vi "Accelerator_v2.001.vi"() -> ()   [LabVIEW 2012]
doc: "Acquire Accelerator Data"
uses:
  <instrlib>/niScope/Controls/niScope vertical coupling.ctl
  <instrlib>/niScope/Controls/niScope trigger slope.ctl
  <instrlib>/niScope/Controls/niScope trigger coupling.ctl
  <instrlib>/niScope/Controls/niScope trigger window mode.ctl
  <instrlib>/niScope/Controls/niScope trigger source.ctl
  Array_Defctl.ctl
  <vilib>/Utility/error.llb/DialogType.ctl
  Database2.0/Public API/Dust_Event.ctl
  Database2.0/Public API/Signal.ctl
  Database2.0/Private/Role ID.ctl
  Database2.0/Private/Hardware ID.ctl
  Database2.0/Private/Estimate_source.ctl
  Database2.0/Private/PSU updated.vi
  <vilib>/addons/database/Connection.llb/Conn Execute.vi
  <vilib>/addons/database/Recordset.llb/Rec Fetch Recordset Data (R).vi
  <vilib>/addons/database/Recordset.llb/Rec Destroy - Connection.vi
  <instrlib>/niScope/Configure/Trigger/niScope Configure Trigger Edge.vi
  <instrlib>/niScope/Configure/Trigger/niScope Configure Trigger Hysteresis.vi
  <instrlib>/niScope/Configure/Trigger/niScope Configure Trigger Window.vi
  <instrlib>/niScope/Configure/Trigger/niScope Configure Trigger Immediate.vi
  <instrlib>/niScope/Acquire/Fetch/niScope Multi Fetch Cluster.vi
  <vilib>/Analysis/baseanly.llb/Mean (DBL).vi
  <vilib>/Utility/file.llb/Write To Spreadsheet File (string).vi
  <vilib>/addons/database/_DB Variant To Data/Database Variant To Data.xnode
  <vilib>/Analysis/NI_AALBase.lvlib
  <vilib>/addons/database/NI_Database_API.lvlib
panel:
  out "?":cluster{dbl, dbl}(knob)={0.0549, 2.0} scale=10.0..0.01
  in  "Ideal Time (Cursor)":dbl=2.0 step=0.01 format="%_2f"
  out "Time Between Triggers":dbl
  out "Average Frequency":dbl format="%#_4g"
  in  "Write to Database?":bool=TRUE
  out "output cluster":T1
  out "error out 4":errorcluster
  out "error out 3":errorcluster
  out "# elements in queue":i32
  out "Stop condition":bool=TRUE
  in  "Limit":dbl
  in  "Limit Triggers":bool
  out "Metadata Path":path=path "G:/default/20120619111009.csv"
  out "created path":path=path "G:/default"
  in  "Write Metadata?":bool
  out "Acquisition #":i32
  out "Numeric":i32=92364
  out "error out 2":errorcluster
  out "Calibration":dbl=24700000000000.0
  in  "WFM Tag":string="trace"
  in  "Location":string="G:\\default"
  in  "Write Raw File?":bool
  out "Saving Raw File...":path=path "G:/2012_06_13_verify_timestamp_labview/trace00000"
  out "Array":T2=["Dev1", "Dev2"]
  in  "Debug Mode\n(Confusing)":bool
  out "Mass":dbl format="%#_3g"
  out "Multi Plot 2":cluster{dbl[], dbl[]}(graph) caption="Multi Plot"
  in  "Acceleration Voltage (MV)":dbl=2.0 format="%_2g"
  out "Charge":dbl format="%#_3g"
  out "Velocity (Est.)":dbl format="%#_6f"
  out "Final Detector (CH3)":waveform(dbl)(graph)={"t0"=timestamp(0 s since 1904-01-01), "dt"=1e-07, "Y"=[]}
  out "Charge Detector/PSU gate (CH2)":waveform(dbl)(graph)={"t0"=timestamp(0 s since 1904-01-01), "dt"=1e-07, "Y"=[]}
  out "Velocity Detectors (CH0 & CH1)":waveform(dbl)[](graph)
  out "Actual Sample Rate":dbl=10000000.0 format="%.0p"
  in  "Reference Position (%)":dbl=40.0 caption="Ref Position" format="%.1f"
  in  "Trigger":T3(tab)=enum."Edge"
  in  "Trigger Source Edge 2":T4="2" caption="Source"
  in  "Trigger Source Edge":T4="0" caption="Source"
  in  "Coupling":T5=1 items=["AC"=0, "DC"=1, "HF Reject"=3, "LF Reject"=4, "AC Plus HF Reject"=1001]
  in  "Slope":T6 caption="Trigger Slope"
  in  "Level":dbl=1.0 caption="Trigger Level" step=0.001 format="%.3f"
  in  "Delay":dbl caption="Trigger Delay" format="%.4p"
  in  "Trigger Source Window 2":T4="0" caption="Source"
  in  "Trigger Source Window":T4="0" caption="Source"
  in  "Window Mode":T7=1
  in  "Delay":dbl caption="Trigger Delay" format="%.4f"
  in  "Low Level":dbl=-0.12 format="%.2f"
  in  "High Level":dbl format="%.2f"
  in  "Window Coupling":T5=1 caption="Coupling" items=["AC"=0, "DC"=1, "HF Reject"=3, "LF Reject"=4, "AC Plus HF Reject"=1001]
  in  "Hysteresis Source Trigger 2":T4="3" caption="Source"
  in  "Hysteresis Source Trigger":T4="1" caption="Source"
  in  "Hysteresis":dbl format="%.2f"
  in  "Delay":dbl caption="Trigger Delay" format="%.4f"
  in  "Slope":T6 caption="Trigger Slope"
  in  "Hysteresis Coupling":T5=1 caption="Coupling" items=["AC"=0, "DC"=1, "HF Reject"=3, "LF Reject"=4, "AC Plus HF Reject"=1001]
  in  "Level":dbl=0.05 caption="Trigger Level" format="%.2f"
  in  "Vertical Coupling":T8=1 items=["AC", "DC", "Ground"]
  in  "Probe Attenuation":dbl=1.0 format="%.1f"
  in  "Vertical Offset":dbl format="%.4f"
  in  "Vertical Range":dbl=5.0 caption="Vertical Range (V)" format="%.2f"
  in  "Bandwidth":dbl=-1.0 format="%.2f"
  in  "Min Record Length":i32=100000 caption="Min. Record Length"
  in  "Min Sample Rate":dbl=80000000.0 caption="Min. Sample Rate" step=1000000.0 format="%.2p"
  out "Actual Record Length":i32=100000
  in  "stop":bool=TRUE
  out "error out":errorcluster={"status"=FALSE, "code"=0, "source"="No Error"} {"code" format="%.0x"}
  # "File Parameters"
  # "Error Handling"
  # "Horizontal"
  # "Vertical"
  # "Channel"
  # "Trigger"
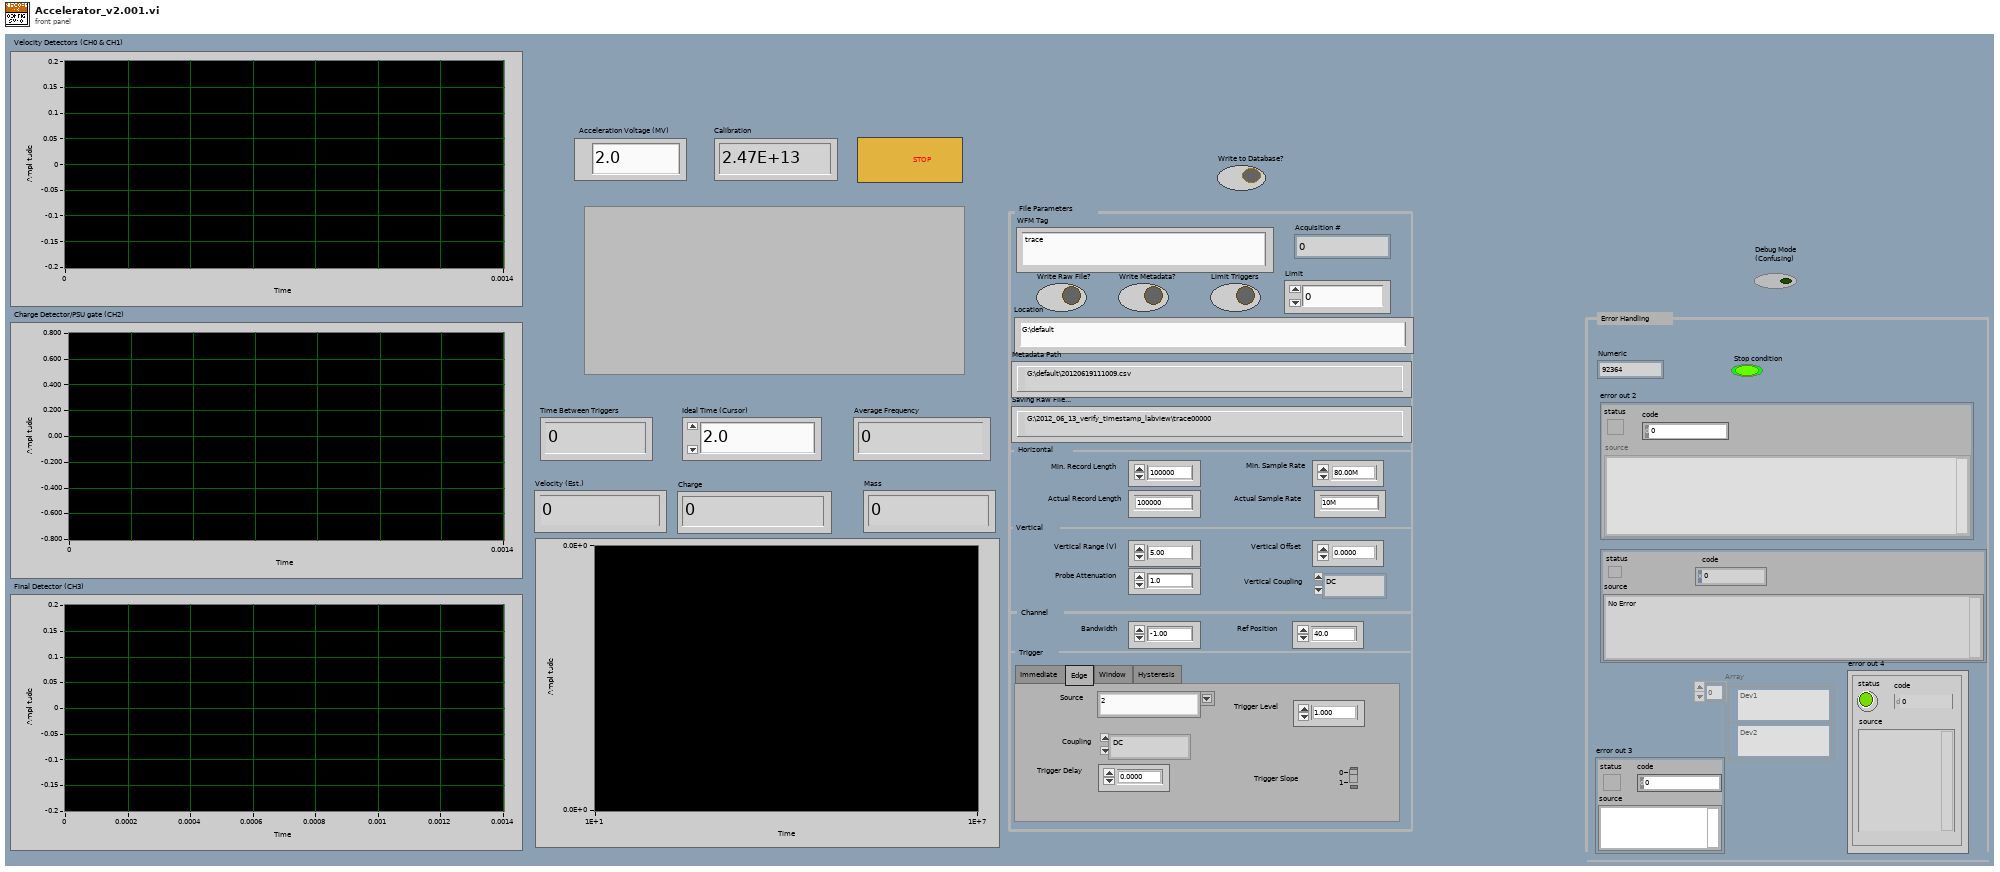
[diagram p1: front panel]
types:
  T1 = cluster{"File Path Control":path, "Array":waveform(dbl)[]}
  T2 = typedef "Array_Defctl.ctl" = refnum<k15>[]
  T3 = enum32{"Immediate", "Edge", "Window", "Hysteresis"}
  T4 = typedef "niScope trigger source.ctl" = string
  T5 = typedef "niScope trigger coupling.ctl" = u16
  T6 = typedef "niScope trigger slope.ctl" = i32
  T7 = typedef "niScope trigger window mode.ctl" = i32
  T8 = typedef "niScope vertical coupling.ctl" = i32
  T9 = typedef "DialogType.ctl" = u16
  T10 = typedef "NI_Database_API.lvlib/Conn ObjectReference.ctl" = refnum<k1>
  T11 = typedef "NI_Database_API.lvlib/Rec ObjectReference.ctl" = refnum<k1>
  T12 = cluster{"Integer Timestamp":dbl, "Max Velocity":dbl, "Min Velocity":dbl}
  T13 = cluster{"first point time":dbl, "xIncrement":dbl, "Waveforms":dbl[]}[]
  T14 = typedef "Dust_Event.ctl" = cluster{"Time Stamp":timestamp, "Velocity":sgl, "Mass":sgl, "Charge":sgl, "Radius":sgl, "Array":T15[], "Dust Event ID":i64, "Passed_3rd_Detector":bool, "Estimate Source":T18, "Estimate Quality":sgl}
  T15 = typedef "Signal.ctl" = cluster{"Signal ID":i64, "Time Stamp":timestamp, "Dust Event ID":i64, "Role ID":T16, "Data":sgl[], "Signal Length":i32, "dt":sgl, "Offset":dbl, "Hardware ID":T17}
  T16 = typedef "Role ID.ctl" = enum16{"First_Detector", "Second_Detector", "Third_Detector", "LeCroy_CH1", "LeCroy_CH2", "LeCroy_CH3", "LeCroy_CH4", "PSU"}
  T17 = typedef "Hardware ID.ctl" = enum16{"Unknown", "CSA 1", "CSA 2", "CSA 3", "CSA 4", "CSA 5", "CSA 6"}
  T18 = typedef "Estimate_source.ctl" = i8
  T19 = cluster{"relativeInitialX":dbl, "xIncrement":dbl, "wfm":dbl[]}[]
  T20 = cluster{"first point time":dbl, "xIncrement":dbl, "Waveforms":dbl[]}
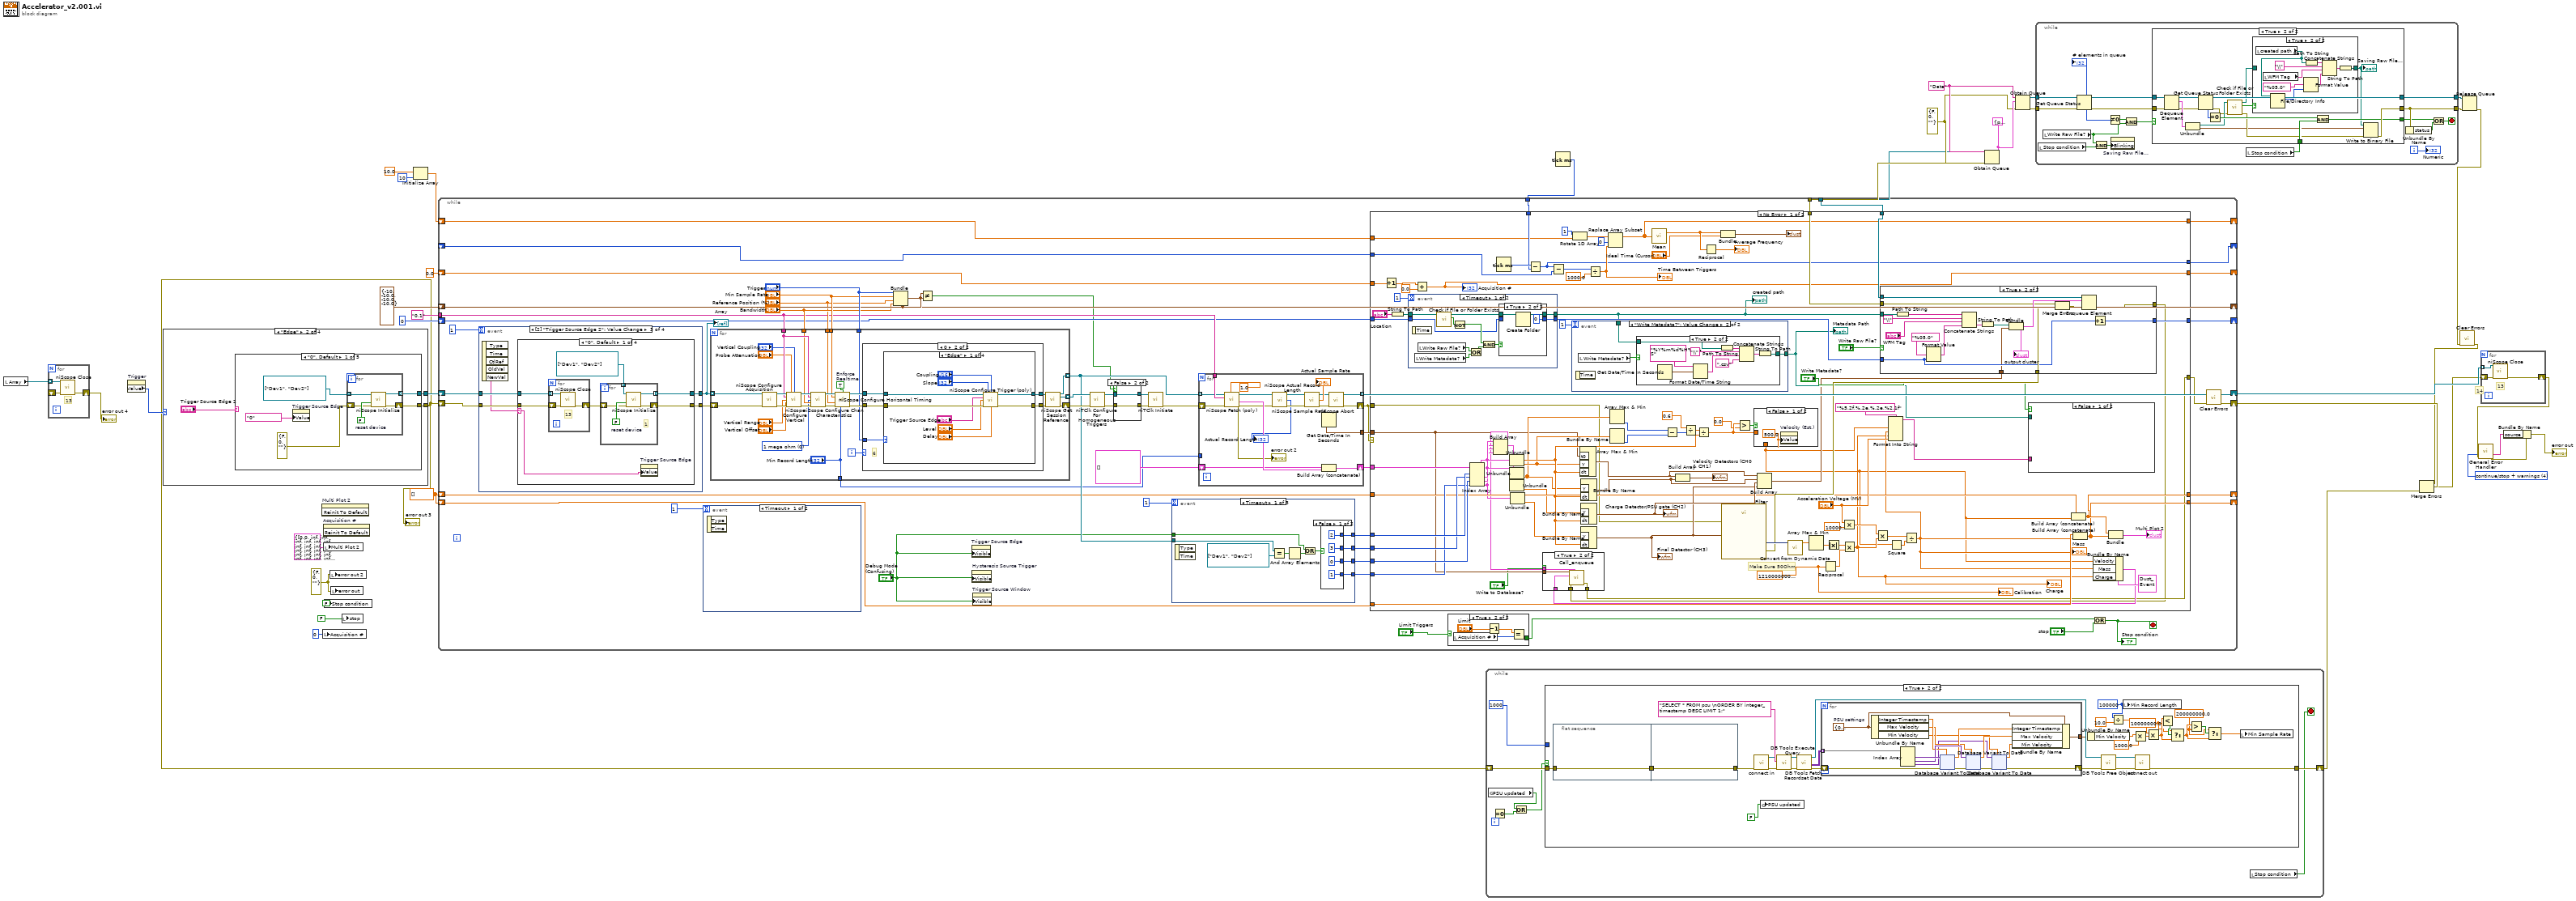
[diagram p0: block diagram]
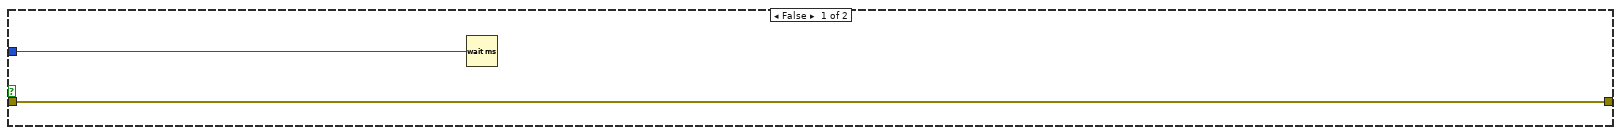
[diagram p2: hidden frame]
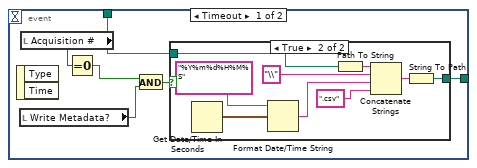
[diagram p4: hidden frame]
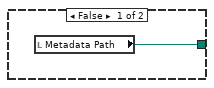
[diagram p5: hidden frame]
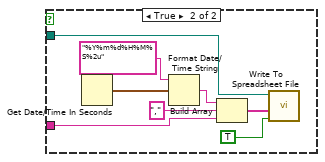
[diagram p7: hidden frame]
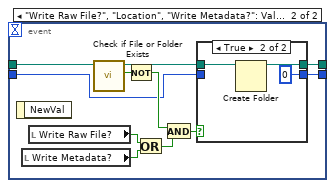
[diagram p9: hidden frame]
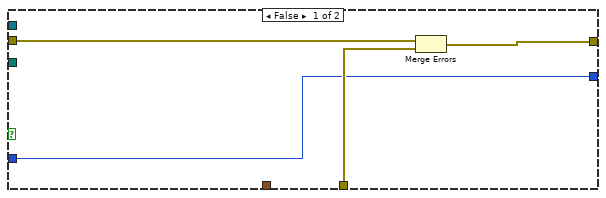
[diagram p11: hidden frame]
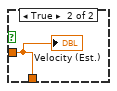
[diagram p12: hidden frame]
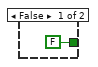
[diagram p14: hidden frame]
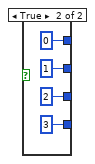
[diagram p15: hidden frame]
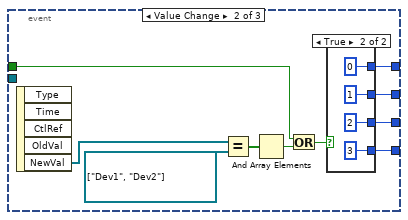
[diagram p16: hidden frame]
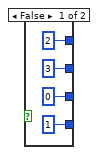
[diagram p17: hidden frame]
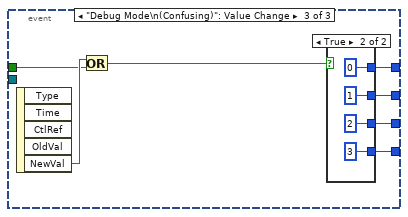
[diagram p18: hidden frame]
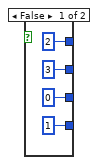
[diagram p19: hidden frame]
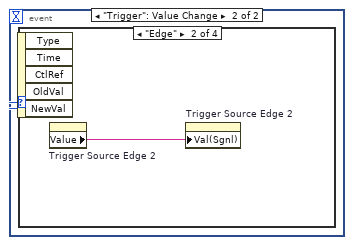
[diagram p20: hidden frame]
diagram:
  w4 = dbl[] []
  w11 = errorcluster {"status"=FALSE, "code"=0, "source"=""} ("error out")
  w16 = errorcluster {"status"=FALSE, "code"=0, "source"=""} ("error out")
  w17 = cluster{path, waveform(sgl)[]} {path "", []} ("output cluster")
  w18 = "Data" ("name (unnamed)")
  w9 = T9 4 items=["no dialog", "OK message", "continue or stop message", "OK message + warnings", "continue/stop + warnings"] ("type of dialog (OK msg:1)")
  # "14"
  n1 = local read "Array"() -> (w19:T2)
  n2 = for {
    tunnel: w19 -> [w40] mode=indexing
    shift-right: [w42] -> w14
    shift-left: _ -> [w41]
    # "13"
    n3 = call <instrlib>:"niScope Close.vi"("instrument handle"=w40, "error in"=w41) -> ("error out"=w42:errorcluster)  [unwired: 13 in]
  }
  "error out 4" <- w14
  n4 = property on="Trigger" class="TabCtl (strict)"() -> ("Value"=w28:T3)  [unwired: 2 in, 2 out]
  n5 = case shown="\"Edge\"" w28 {
    tunnel: [w44 w54 w107 w150] -> w38
    tunnel: [w43 w53 w106 w149] -> w2
    frame "Immediate", Default {
      n6 = for {
        tunnel: refnum<k15>[] ["Dev1", "Dev2"] ("Resources") -> [w50] mode=indexing
        tunnel: [w48] -> w44 mode=indexing
        shift-right: [w47] -> w43
        shift-left: errorcluster {"status"=FALSE, "code"=0, "source"=""} ("error out") -> [w49]
        w51 = FALSE  # reset device
        n7 = call <instrlib>:"niScope Initialize.vi"("resource name"=w50, "reset device"=w51, "error in"=w49) -> ("instrument handle"=w48:refnum<k15>, "error out"=w47:errorcluster)  [unwired: 11 in]
      }
    }
    frame "Edge" {
      n8 = case shown="\"0\", Default" "Trigger Source Edge 2" {
        tunnel: [w59 w67 w77 w87 w99] -> w54
        tunnel: [w58 w66 w76 w86 w98] -> w53
        frame "0", Default {
          n9 = property on="Trigger Source Edge" class="CmbBox (strict)"("Value"=T4 "0" ("Trigger Source Edge")) -> ()  [unwired: 2 in, 2 out]
          n10 = for {
            tunnel: refnum<k15>[] ["Dev1", "Dev2"] ("Resources") -> [w63] mode=indexing
            tunnel: [w61] -> w59 mode=indexing
            shift-right: [w60] -> w58
            shift-left: errorcluster {"status"=FALSE, "code"=0, "source"=""} ("error out") -> [w62]
            w64 = FALSE  # reset device
            n11 = call <instrlib>:"niScope Initialize.vi"("resource name"=w63, "reset device"=w64, "error in"=w62) -> ("instrument handle"=w61:refnum<k15>, "error out"=w60:errorcluster)  [unwired: 11 in]
          }
        }
        frame "1" {
          n12 = property on="Trigger Source Edge" class="CmbBox (strict)"("Value"=T4 "1" ("Trigger Source Edge")) -> ()  [unwired: 2 in, 2 out]
          n13 = for {
            tunnel: refnum<k15>[] ["Dev1", "Dev2"] ("Resources") -> [w73] mode=indexing
            tunnel: [w71] -> w67 mode=indexing
            shift-right: [w70] -> w66
            shift-left: errorcluster {"status"=FALSE, "code"=0, "source"=""} ("error out") -> [w72]
            w74 = FALSE  # reset device
            # "1"
            n14 = call <instrlib>:"niScope Initialize.vi"("resource name"=w73, "reset device"=w74, "error in"=w72) -> ("instrument handle"=w71:refnum<k15>, "error out"=w70:errorcluster)  [unwired: 11 in]
          }
        }
        frame "2" {
          n15 = property on="Trigger Source Edge" class="CmbBox (strict)"("Value"=T4 "0" ("Trigger Source Edge")) -> ()  [unwired: 2 in, 2 out]
          n16 = for {
            tunnel: refnum<k15>[] ["Dev2", "Dev1"] ("Resources") -> [w83] mode=indexing
            tunnel: [w81] -> w77 mode=indexing
            shift-right: [w80] -> w76
            shift-left: errorcluster {"status"=FALSE, "code"=0, "source"=""} ("error out") -> [w82]
            w84 = FALSE  # reset device
            # "1"
            n17 = call <instrlib>:"niScope Initialize.vi"("resource name"=w83, "reset device"=w84, "error in"=w82) -> ("instrument handle"=w81:refnum<k15>, "error out"=w80:errorcluster)  [unwired: 11 in]
          }
        }
        frame "3" {
          n18 = property on="Trigger Source Edge" class="CmbBox (strict)"("Value"=T4 "1" ("Trigger Source Edge")) -> ()  [unwired: 2 in, 2 out]
          n19 = for {
            tunnel: refnum<k15>[] ["Dev2", "Dev1"] ("Resources") -> [w93] mode=indexing
            tunnel: [w91] -> w87 mode=indexing
            shift-right: [w90] -> w86
            shift-left: errorcluster {"status"=FALSE, "code"=0, "source"=""} ("error out") -> [w92]
            w94 = FALSE  # reset device
            # "1"
            n20 = call <instrlib>:"niScope Initialize.vi"("resource name"=w93, "reset device"=w94, "error in"=w92) -> ("instrument handle"=w91:refnum<k15>, "error out"=w90:errorcluster)  [unwired: 11 in]
          }
        }
        frame "VAL_EXTERNAL" {
          n21 = property on="Trigger Source Edge" class="CmbBox (strict)"("Value"=T4 "VAL_EXTERNAL" ("Trigger Source Edge")) -> ()  [unwired: 2 in, 2 out]
          n22 = for {
            tunnel: refnum<k15>[] ["Dev1", "Dev2"] ("Resources") -> [w103] mode=indexing
            tunnel: [w101] -> w99 mode=indexing
            shift-right: [w100] -> w98
            shift-left: errorcluster {"status"=FALSE, "code"=0, "source"=""} ("error out") -> [w102]
            w104 = FALSE  # reset device
            n23 = call <instrlib>:"niScope Initialize.vi"("resource name"=w103, "reset device"=w104, "error in"=w102) -> ("instrument handle"=w101:refnum<k15>, "error out"=w100:errorcluster)  [unwired: 11 in]
          }
        }
      }
    }
    frame "Window" {
      n24 = case shown="\"3\"" "Trigger Source Window 2" {
        tunnel: [w112 w120 w130 w140] -> w107
        tunnel: [w111 w119 w129 w139] -> w106
        frame "0", Default {
          n25 = property on="Trigger Source Window" class="CmbBox (strict)"("Value"=T4 "0" ("Trigger Source Edge")) -> ()  [unwired: 2 in, 2 out]
          n26 = for {
            tunnel: refnum<k15>[] ["Dev1", "Dev2"] ("Resources") -> [w116] mode=indexing
            tunnel: [w114] -> w112 mode=indexing
            shift-right: [w113] -> w111
            shift-left: errorcluster {"status"=FALSE, "code"=0, "source"=""} ("error out") -> [w115]
            w117 = FALSE  # reset device
            # "1"
            n27 = call <instrlib>:"niScope Initialize.vi"("resource name"=w116, "reset device"=w117, "error in"=w115) -> ("instrument handle"=w114:refnum<k15>, "error out"=w113:errorcluster)  [unwired: 11 in]
          }
        }
        frame "1" {
          n28 = property on="Trigger Source Window" class="CmbBox (strict)"("Value"=T4 "1" ("Trigger Source Edge")) -> ()  [unwired: 2 in, 2 out]
          n29 = for {
            tunnel: refnum<k15>[] ["Dev1", "Dev2"] ("Resources") -> [w126] mode=indexing
            tunnel: [w124] -> w120 mode=indexing
            shift-right: [w123] -> w119
            shift-left: errorcluster {"status"=FALSE, "code"=0, "source"=""} ("error out") -> [w125]
            w127 = FALSE  # reset device
            # "1"
            n30 = call <instrlib>:"niScope Initialize.vi"("resource name"=w126, "reset device"=w127, "error in"=w125) -> ("instrument handle"=w124:refnum<k15>, "error out"=w123:errorcluster)  [unwired: 11 in]
          }
        }
        frame "2" {
          n31 = property on="Trigger Source Window" class="CmbBox (strict)"("Value"=T4 "0" ("Trigger Source Edge")) -> ()  [unwired: 2 in, 2 out]
          n32 = for {
            tunnel: refnum<k15>[] ["Dev2", "Dev1"] ("Resources") -> [w136] mode=indexing
            tunnel: [w134] -> w130 mode=indexing
            shift-right: [w133] -> w129
            shift-left: errorcluster {"status"=FALSE, "code"=0, "source"=""} ("error out") -> [w135]
            w137 = FALSE  # reset device
            # "1"
            n33 = call <instrlib>:"niScope Initialize.vi"("resource name"=w136, "reset device"=w137, "error in"=w135) -> ("instrument handle"=w134:refnum<k15>, "error out"=w133:errorcluster)  [unwired: 11 in]
          }
        }
        frame "3" {
          n34 = property on="Trigger Source Window" class="CmbBox (strict)"("Value"=T4 "1" ("Trigger Source Edge")) -> ()  [unwired: 2 in, 2 out]
          n35 = for {
            tunnel: refnum<k15>[] ["Dev2", "Dev1"] ("Resources") -> [w146] mode=indexing
            tunnel: [w144] -> w140 mode=indexing
            shift-right: [w143] -> w139
            shift-left: errorcluster {"status"=FALSE, "code"=0, "source"=""} ("error out") -> [w145]
            w147 = FALSE  # reset device
            # "1"
            n36 = call <instrlib>:"niScope Initialize.vi"("resource name"=w146, "reset device"=w147, "error in"=w145) -> ("instrument handle"=w144:refnum<k15>, "error out"=w143:errorcluster)  [unwired: 11 in]
          }
        }
      }
    }
    frame "Hysteresis" {
      n37 = case shown="\"1\"" "Hysteresis Source Trigger 2" {
        selector: "Hysteresis Source Trigger 2" -> [w151 w161 _ _]
        tunnel: [w155 w163 w173 w183] -> w150
        tunnel: [w154 w162 w172 w182] -> w149
        frame "0", Default {
          n38 = property on="Hysteresis Source Trigger" class="CmbBox (strict)"("Value"=w151) -> ()  [unwired: 2 in, 2 out]
          n39 = for {
            tunnel: refnum<k15>[] ["Dev1", "Dev2"] ("Resources") -> [w159] mode=indexing
            tunnel: [w157] -> w155 mode=indexing
            shift-right: [w156] -> w154
            shift-left: errorcluster {"status"=FALSE, "code"=0, "source"=""} ("error out") -> [w158]
            w160 = FALSE  # reset device
            # "1"
            n40 = call <instrlib>:"niScope Initialize.vi"("resource name"=w159, "reset device"=w160, "error in"=w158) -> ("instrument handle"=w157:refnum<k15>, "error out"=w156:errorcluster)  [unwired: 11 in]
          }
        }
        frame "1" {
          n41 = property on="Hysteresis Source Trigger" class="CmbBox (strict)"("Value"=w161) -> ()  [unwired: 2 in, 2 out]
          n42 = for {
            tunnel: refnum<k15>[] ["Dev1", "Dev2"] ("Resources") -> [w169] mode=indexing
            tunnel: [w167] -> w163 mode=indexing
            shift-right: [w166] -> w162
            shift-left: errorcluster {"status"=FALSE, "code"=0, "source"=""} ("error out") -> [w168]
            w170 = FALSE  # reset device
            # "1"
            n43 = call <instrlib>:"niScope Initialize.vi"("resource name"=w169, "reset device"=w170, "error in"=w168) -> ("instrument handle"=w167:refnum<k15>, "error out"=w166:errorcluster)  [unwired: 11 in]
          }
        }
        frame "2" {
          n44 = property on="Hysteresis Source Trigger" class="CmbBox (strict)"("Value"=T4 "0" ("Trigger Source Edge")) -> ()  [unwired: 2 in, 2 out]
          n45 = for {
            tunnel: refnum<k15>[] ["Dev2", "Dev1"] ("Resources") -> [w179] mode=indexing
            tunnel: [w177] -> w173 mode=indexing
            shift-right: [w176] -> w172
            shift-left: errorcluster {"status"=FALSE, "code"=0, "source"=""} ("error out") -> [w178]
            w180 = FALSE  # reset device
            # "1"
            n46 = call <instrlib>:"niScope Initialize.vi"("resource name"=w179, "reset device"=w180, "error in"=w178) -> ("instrument handle"=w177:refnum<k15>, "error out"=w176:errorcluster)  [unwired: 11 in]
          }
        }
        frame "3" {
          n47 = property on="Hysteresis Source Trigger" class="CmbBox (strict)"("Value"=T4 "1" ("Trigger Source Edge")) -> ()  [unwired: 2 in, 2 out]
          n48 = for {
            tunnel: refnum<k15>[] ["Dev2", "Dev1"] ("Resources") -> [w189] mode=indexing
            tunnel: [w187] -> w183 mode=indexing
            shift-right: [w186] -> w182
            shift-left: errorcluster {"status"=FALSE, "code"=0, "source"=""} ("error out") -> [w188]
            w190 = FALSE  # reset device
            # "1"
            n49 = call <instrlib>:"niScope Initialize.vi"("resource name"=w189, "reset device"=w190, "error in"=w188) -> ("instrument handle"=w187:refnum<k15>, "error out"=w186:errorcluster)  [unwired: 11 in]
          }
        }
      }
    }
  }
  "error out 3" <- w2
  n50 = invoke on="Multi Plot 2" class="XYGraph (strict)" method="Reinit To Default"() -> ()  [unwired: 3 in, 3 out]
  n51 = local write "Acquisition #"(0 ("Acquisition #")) -> ()
  n52 = invoke on="Acquisition #" class="DigNum (strict)" method="Reinit To Default"() -> ()  [unwired: 3 in, 3 out]
  n53 = local write "Multi Plot 2"(cluster{dbl[], dbl[]} {[0.0, inf, inf, inf, inf, inf, inf, inf, inf, inf, inf, inf, inf, inf, inf, inf, inf, inf, inf, inf, inf, inf, inf, inf, inf, inf, inf, inf, inf, inf, inf, inf, inf, inf, inf, inf, inf, inf, inf, inf, inf], [0.0, 0.0, 0.0, 0.0, 0.0, 0.0, 0.0, 0.0, 0.0, 0.0, 0.0, 0.0, 0.0, 0.0, 0.0, 0.0, 0.0, 0.0, 0.0, 0.0, 0.0, 0.0, 0.0, 0.0, 0.0, 0.0, 0.0, 0.0, 0.0, 0.0, 0.0, 0.0, 0.0, 0.0, 0.0, 0.0, 0.0, 0.0, 0.0, 0.0, 0.0]} ("Multi Plot 2")) -> ()
  n54 = local write "Stop condition"(FALSE ("x .or. y?")) -> ()
  n55 = local write "error out 2"(w11) -> ()
  n56 = local write "error out"(w11) -> ()
  n57 = local write "stop"(FALSE ("stop")) -> ()
  n58 = Initialize Array(10.0 ("element"), 10 ("dimension size")) -> (w30:dbl[])
  n59 = while {
    shift-right: [w197] -> w1
    shift-left: w2 -> [w198]
    i -> [w196]
    stop <- w195 stop-if-true
    n60 = global read "PSU updated.vi" "PSU updated"() -> (w194:bool)
    n61 = Equal To 0?(x=w196) -> (x = 0?=w192:bool)
    n62 = Or(x=w194, y=w192) -> (x .or. y?=w193:bool)
    n63 = case shown="True" w193 {
      tunnel: w198 -> [w199 w229]
      tunnel: [w199 w228] -> w197
      tunnel: 1000 -> [w200 _]
      frame False {
        n64 = Wait (ms)(milliseconds to wait=w200) -> ()  [unwired: 1 out]
      }
      frame True {
        w202 = 200000000.0 ("y")
        w205 = 10000000.0 ("y")
        w212 = 100000 ("Min Record Length")
        n65 = flat-sequence {
          tunnel: [w231] -> w230
          tunnel: w229 -> [w231]
          tunnel: w230 -> [w232]
          tunnel: [w232] -> w215
          frame #0 {
          }
          frame #1 {
          }
        }
        n66 = call "connect in.vi"("error in (no error)"=w215) -> ("error out"=w219:errorcluster, "Database Connection"=w218:T10)  [unwired: 6 in, 1 out]
        n67 = global write "PSU updated.vi" "PSU updated"(FALSE ("PSU updated")) -> ()
        n68 = call-poly <vilib>:"DB Tools Execute Query.vi"("error in (no error)"=w219, "SQL query"="SELECT * FROM psu \nORDER BY integer_timestamp DESC LIMIT 1;", "connection reference"=w218) -> ("error out"=w221:errorcluster, "recordset reference"=w220:T11)  [unwired: 5 in]
        n69 = call-poly <vilib>:"DB Tools Fetch Recordset Data.vi"("error in (no error)"=w221, "recordset reference"=w220) -> ("error out"=w227:errorcluster, "recordset data"=w226:variant[][], "recordset reference out"=w222:T11)  [unwired: 3 in]
        n70 = for {
          tunnel: w226 -> [w248] mode=indexing
          shift-right: [w233] -> w216
          shift-left: w227 -> [w244]
          tunnel: [w243] -> w217
          w238 = T12 {"Integer Timestamp"=0.0, "Max Velocity"=0.0, "Min Velocity"=0.0}  # PSU settings
          n71 = Unbundle By Name(w238) -> ("Integer Timestamp"=w242:dbl, "Max Velocity"=w239:dbl, "Min Velocity"=w236:dbl)
          n72 = Index Array(array=w248) -> (element #1=w247:variant, element #2=w246:variant, element #3=w237:variant)  [unwired: 3 in]
          n73 = xnode "Database Variant To Data"("database variant"=w247, "error in"=w244, "type"=w242) -> ("data"=w241:dbl, "error out"=w245:errorcluster)
          n74 = xnode "Database Variant To Data"("database variant"=w246, "error in"=w245, "type"=w239) -> ("data"=w240:dbl, "error out"=w234:errorcluster)
          n75 = xnode "Database Variant To Data"("database variant"=w237, "error in"=w234, "type"=w236) -> ("data"=w235:dbl, "error out"=w233:errorcluster)
          n76 = Bundle By Name(cluster=w238, "Integer Timestamp"=w241, "Max Velocity"=w240, "Min Velocity"=w235) -> (w243:T12)
        }
        n77 = Unbundle By Name(w217) -> ("Min Velocity"=w211:dbl)
        n78 = call-poly <vilib>:"DB Tools Free Object.vi"("error in (no error)"=w216, "recordset reference"=w222) -> ("error out"=w223:errorcluster, "connection reference"=w224:T10)  [unwired: 8 in]
        n79 = Divide(x=w212, y=10.0) -> (x/y=w208:dbl)
        n80 = local write "Min Record Length"(w212) -> ()
        n81 = Multiply(x=w211, y=1000.0) -> (x*y=w209:dbl)
        n82 = call "connect out.vi"("error in (no error)"=w223, "connection reference"=w224) -> ("error out"=w228:errorcluster)  [unwired: 9 in]
        n83 = Multiply(x=w208, y=w209) -> (x*y=w206:dbl)
        n84 = Less?(x=w206, y=w205) -> (x < y?=w207:bool)
        n85 = Select(t=w205, s=w207, f=w206) -> (s? t:f=w204:dbl)
        n86 = Greater?(x=w204, y=w202) -> (0:w203:bool)
        n87 = Select(t=w202, s=w203, f=w204) -> (s? t:f=w201:dbl)
        n88 = local write "Min Sample Rate"(w201) -> ()
      }
    }
    n89 = local read "Stop condition"() -> (w195:bool)
  }
  n90 = Tick Count (ms)() -> (millisecond timer value=w33:u32)
  n91 = Obtain Queue(name (unnamed)=w18, element data type=w17, error in (no error)=w16) -> (queue out=w13:refnum<queue>, error out=w26:errorcluster)  [unwired: 2 in, 1 out]
  n92 = while {
    shift-right: [w353] -> w12
    shift-left: w2 -> [w358]
    shift-right: [w392] -> _
    shift-left: cluster{i32, dbl, dbl, dbl} {-10, -10.0, -10.0, -10.0} -> [w393]
    tunnel: w33 -> [w350]
    shift-right: [w348] -> _
    shift-left: w30 -> [w349]
    shift-right: [w347] -> _
    shift-left: _ -> [w351]
    shift-right: [w385] -> _
    shift-left: w4 -> [w362]
    shift-right: [w384] -> _
    shift-left: w4 -> [w383]
    tunnel: "0,1" ("Channel Name") -> [w382]
    shift-right: [w359] -> w27
    shift-left: w38 -> [w380]
    tunnel: w13 -> [w369]
    tunnel: w26 -> [w368]
    shift-right: [w367] -> _
    shift-left: 0 -> [w366]
    shift-right: [w345] -> _
    shift-left: 0.0 -> [w346]
    stop <- w357 stop-if-true
    n93 = event shown="[2] \"Trigger Source Edge 2\": Value Change" {
      selector: _ -> [_ _ _ _]
      dyn-events: _ -> [_ _ _ _]
      timeout: 1 -> [_ _ _ _]
      tunnel: w380 -> [w675 w680 w744 w810]
      tunnel: [w675 w679 w742 w808] -> w377
      tunnel: w358 -> [w674 w678 w745 w809]
      tunnel: [w674 w677 w741 w807] -> w378
      event Timeout {
        n94 = event-data() -> ()  [unwired: 1 in, 2 out]
      }
      event Value Change {
        n95 = event-data() -> ("NewVal"=w676:T4)  [unwired: 1 in, 4 out]
        n96 = case shown="\"1\"" w676 {
          selector: w676 -> [w687 w702 _ _]
          tunnel: w680 -> [w682 w697 w715 w728]
          tunnel: [w684 w699 w713 w729] -> w679
          tunnel: w678 -> [w681 w696 w714 w727]
          tunnel: [w683 w698 w712 w730] -> w677
          frame "0", Default {
            n97 = for {
              tunnel: w682 -> [w688] mode=indexing
              shift-right: [w690] -> w685
              shift-left: w681 -> [w689]
              n98 = call <instrlib>:"niScope Close.vi"("instrument handle"=w688, "error in"=w689) -> ("error out"=w690:errorcluster)  [unwired: 13 in]
            }
            n99 = for {
              tunnel: [w694] -> w684 mode=indexing
              shift-right: [w693] -> w683
              shift-left: w685 -> [w691]
              tunnel: refnum<k15>[] ["Dev1", "Dev2"] ("Resources") -> [w692] mode=indexing
              w695 = FALSE  # reset device
              n100 = call <instrlib>:"niScope Initialize.vi"("resource name"=w692, "reset device"=w695, "error in"=w691) -> ("instrument handle"=w694:refnum<k15>, "error out"=w693:errorcluster)  [unwired: 11 in]
            }
            n101 = property on="Hysteresis Source Trigger" class="CmbBox (strict)"("Value"=w687) -> ()  [unwired: 2 in, 2 out]
          }
          frame "1" {
            n102 = for {
              tunnel: w697 -> [w703] mode=indexing
              shift-right: [w705] -> w700
              shift-left: w696 -> [w704]
              n103 = call <instrlib>:"niScope Close.vi"("instrument handle"=w703, "error in"=w704) -> ("error out"=w705:errorcluster)  [unwired: 13 in]
            }
            n104 = for {
              tunnel: [w709] -> w699 mode=indexing
              shift-right: [w708] -> w698
              shift-left: w700 -> [w706]
              tunnel: refnum<k15>[] ["Dev1", "Dev2"] ("Resources") -> [w707] mode=indexing
              w710 = FALSE  # reset device
              n105 = call <instrlib>:"niScope Initialize.vi"("resource name"=w707, "reset device"=w710, "error in"=w706) -> ("instrument handle"=w709:refnum<k15>, "error out"=w708:errorcluster)  [unwired: 11 in]
            }
            n106 = property on="Hysteresis Source Trigger" class="CmbBox (strict)"("Value"=w702) -> ()  [unwired: 2 in, 2 out]
          }
          frame "2" {
            n107 = for {
              tunnel: w715 -> [w718] mode=indexing
              shift-right: [w720] -> w716
              shift-left: w714 -> [w719]
              # "13"
              n108 = call <instrlib>:"niScope Close.vi"("instrument handle"=w718, "error in"=w719) -> ("error out"=w720:errorcluster)  [unwired: 13 in]
            }
            n109 = for {
              tunnel: [w724] -> w713 mode=indexing
              shift-right: [w723] -> w712
              shift-left: w716 -> [w721]
              tunnel: refnum<k15>[] ["Dev2", "Dev1"] ("Resources") -> [w722] mode=indexing
              w725 = FALSE  # reset device
              # "1"
              n110 = call <instrlib>:"niScope Initialize.vi"("resource name"=w722, "reset device"=w725, "error in"=w721) -> ("instrument handle"=w724:refnum<k15>, "error out"=w723:errorcluster)  [unwired: 11 in]
            }
            n111 = property on="Hysteresis Source Trigger" class="CmbBox (strict)"("Value"=T4 "0" ("Trigger Source Edge")) -> ()  [unwired: 2 in, 2 out]
          }
          frame "3" {
            n112 = for {
              tunnel: w728 -> [w733] mode=indexing
              shift-right: [w735] -> w731
              shift-left: w727 -> [w734]
              # "13"
              n113 = call <instrlib>:"niScope Close.vi"("instrument handle"=w733, "error in"=w734) -> ("error out"=w735:errorcluster)  [unwired: 13 in]
            }
            n114 = for {
              tunnel: [w739] -> w729 mode=indexing
              shift-right: [w738] -> w730
              shift-left: w731 -> [w736]
              tunnel: refnum<k15>[] ["Dev2", "Dev1"] ("Resources") -> [w737] mode=indexing
              w740 = FALSE  # reset device
              # "1"
              n115 = call <instrlib>:"niScope Initialize.vi"("resource name"=w737, "reset device"=w740, "error in"=w736) -> ("instrument handle"=w739:refnum<k15>, "error out"=w738:errorcluster)  [unwired: 11 in]
            }
            n116 = property on="Hysteresis Source Trigger" class="CmbBox (strict)"("Value"=T4 "1" ("Trigger Source Edge")) -> ()  [unwired: 2 in, 2 out]
          }
        }
      }
      event Value Change {
        n117 = event-data() -> ("NewVal"=w743:T4)  [unwired: 1 in, 4 out]
        n118 = case shown="\"0\", Default" w743 {
          selector: w743 -> [w746 w761 _ _]
          tunnel: w744 -> [w748 w763 w780 w793]
          tunnel: [w750 w765 w778 w794] -> w742
          tunnel: w745 -> [w747 w762 w779 w792]
          tunnel: [w749 w764 w777 w795] -> w741
          frame "0", Default {
            n119 = for {
              tunnel: w748 -> [w753] mode=indexing
              shift-right: [w755] -> w751
              shift-left: w747 -> [w754]
              # "13"
              n120 = call <instrlib>:"niScope Close.vi"("instrument handle"=w753, "error in"=w754) -> ("error out"=w755:errorcluster)  [unwired: 13 in]
            }
            n121 = for {
              tunnel: [w759] -> w750 mode=indexing
              shift-right: [w758] -> w749
              shift-left: w751 -> [w756]
              tunnel: refnum<k15>[] ["Dev1", "Dev2"] ("Resources") -> [w757] mode=indexing
              w760 = FALSE  # reset device
              # "1"
              n122 = call <instrlib>:"niScope Initialize.vi"("resource name"=w757, "reset device"=w760, "error in"=w756) -> ("instrument handle"=w759:refnum<k15>, "error out"=w758:errorcluster)  [unwired: 11 in]
            }
            n123 = property on="Trigger Source Edge" class="CmbBox (strict)"("Value"=w746) -> ()  [unwired: 2 in, 2 out]
          }
          frame "1" {
            n124 = for {
              tunnel: w763 -> [w768] mode=indexing
              shift-right: [w770] -> w766
              shift-left: w762 -> [w769]
              # "13"
              n125 = call <instrlib>:"niScope Close.vi"("instrument handle"=w768, "error in"=w769) -> ("error out"=w770:errorcluster)  [unwired: 13 in]
            }
            n126 = for {
              tunnel: [w774] -> w765 mode=indexing
              shift-right: [w773] -> w764
              shift-left: w766 -> [w771]
              tunnel: refnum<k15>[] ["Dev1", "Dev2"] ("Resources") -> [w772] mode=indexing
              w775 = FALSE  # reset device
              # "1"
              n127 = call <instrlib>:"niScope Initialize.vi"("resource name"=w772, "reset device"=w775, "error in"=w771) -> ("instrument handle"=w774:refnum<k15>, "error out"=w773:errorcluster)  [unwired: 11 in]
            }
            n128 = property on="Trigger Source Edge" class="CmbBox (strict)"("Value"=w761) -> ()  [unwired: 2 in, 2 out]
          }
          frame "2" {
            n129 = for {
              tunnel: w780 -> [w783] mode=indexing
              shift-right: [w785] -> w781
              shift-left: w779 -> [w784]
              # "13"
              n130 = call <instrlib>:"niScope Close.vi"("instrument handle"=w783, "error in"=w784) -> ("error out"=w785:errorcluster)  [unwired: 13 in]
            }
            n131 = for {
              tunnel: [w789] -> w778 mode=indexing
              shift-right: [w788] -> w777
              shift-left: w781 -> [w786]
              tunnel: refnum<k15>[] ["Dev2", "Dev1"] ("Resources") -> [w787] mode=indexing
              w790 = FALSE  # reset device
              # "1"
              n132 = call <instrlib>:"niScope Initialize.vi"("resource name"=w787, "reset device"=w790, "error in"=w786) -> ("instrument handle"=w789:refnum<k15>, "error out"=w788:errorcluster)  [unwired: 11 in]
            }
            n133 = property on="Trigger Source Edge" class="CmbBox (strict)"("Value"=T4 "0" ("Trigger Source Edge")) -> ()  [unwired: 2 in, 2 out]
          }
          frame "3" {
            n134 = for {
              tunnel: w793 -> [w798] mode=indexing
              shift-right: [w800] -> w796
              shift-left: w792 -> [w799]
              # "13"
              n135 = call <instrlib>:"niScope Close.vi"("instrument handle"=w798, "error in"=w799) -> ("error out"=w800:errorcluster)  [unwired: 13 in]
            }
            n136 = for {
              tunnel: [w804] -> w794 mode=indexing
              shift-right: [w803] -> w795
              shift-left: w796 -> [w801]
              tunnel: refnum<k15>[] ["Dev2", "Dev1"] ("Resources") -> [w802] mode=indexing
              w805 = FALSE  # reset device
              # "1"
              n137 = call <instrlib>:"niScope Initialize.vi"("resource name"=w802, "reset device"=w805, "error in"=w801) -> ("instrument handle"=w804:refnum<k15>, "error out"=w803:errorcluster)  [unwired: 11 in]
            }
            n138 = property on="Trigger Source Edge" class="CmbBox (strict)"("Value"=T4 "1" ("Trigger Source Edge")) -> ()  [unwired: 2 in, 2 out]
          }
        }
      }
      event Value Change {
        n139 = event-data() -> ("NewVal"=w806:T4)  [unwired: 1 in, 4 out]
        n140 = case shown="\"1\"" w806 {
          selector: w806 -> [w811 w826 _ _]
          tunnel: w810 -> [w813 w828 w845 w858]
          tunnel: [w815 w830 w843 w859] -> w808
          tunnel: w809 -> [w812 w827 w844 w857]
          tunnel: [w814 w829 w842 w860] -> w807
          frame "0", Default {
            n141 = for {
              tunnel: w813 -> [w818] mode=indexing
              shift-right: [w820] -> w816
              shift-left: w812 -> [w819]
              # "13"
              n142 = call <instrlib>:"niScope Close.vi"("instrument handle"=w818, "error in"=w819) -> ("error out"=w820:errorcluster)  [unwired: 13 in]
            }
            n143 = for {
              tunnel: [w824] -> w815 mode=indexing
              shift-right: [w823] -> w814
              shift-left: w816 -> [w821]
              tunnel: refnum<k15>[] ["Dev1", "Dev2"] ("Resources") -> [w822] mode=indexing
              w825 = FALSE  # reset device
              # "1"
              n144 = call <instrlib>:"niScope Initialize.vi"("resource name"=w822, "reset device"=w825, "error in"=w821) -> ("instrument handle"=w824:refnum<k15>, "error out"=w823:errorcluster)  [unwired: 11 in]
            }
            n145 = property on="Trigger Source Window" class="CmbBox (strict)"("Value"=w811) -> ()  [unwired: 2 in, 2 out]
          }
          frame "1" {
            n146 = for {
              tunnel: w828 -> [w833] mode=indexing
              shift-right: [w835] -> w831
              shift-left: w827 -> [w834]
              # "13"
              n147 = call <instrlib>:"niScope Close.vi"("instrument handle"=w833, "error in"=w834) -> ("error out"=w835:errorcluster)  [unwired: 13 in]
            }
            n148 = for {
              tunnel: [w839] -> w830 mode=indexing
              shift-right: [w838] -> w829
              shift-left: w831 -> [w836]
              tunnel: refnum<k15>[] ["Dev1", "Dev2"] ("Resources") -> [w837] mode=indexing
              w840 = FALSE  # reset device
              # "1"
              n149 = call <instrlib>:"niScope Initialize.vi"("resource name"=w837, "reset device"=w840, "error in"=w836) -> ("instrument handle"=w839:refnum<k15>, "error out"=w838:errorcluster)  [unwired: 11 in]
            }
            n150 = property on="Trigger Source Window" class="CmbBox (strict)"("Value"=w826) -> ()  [unwired: 2 in, 2 out]
          }
          frame "2" {
            n151 = for {
              tunnel: w845 -> [w848] mode=indexing
              shift-right: [w850] -> w846
              shift-left: w844 -> [w849]
              n152 = call <instrlib>:"niScope Close.vi"("instrument handle"=w848, "error in"=w849) -> ("error out"=w850:errorcluster)  [unwired: 13 in]
            }
            n153 = for {
              tunnel: [w854] -> w843 mode=indexing
              shift-right: [w853] -> w842
              shift-left: w846 -> [w851]
              tunnel: refnum<k15>[] ["Dev2", "Dev1"] ("Resources") -> [w852] mode=indexing
              w855 = FALSE  # reset device
              # "1"
              n154 = call <instrlib>:"niScope Initialize.vi"("resource name"=w852, "reset device"=w855, "error in"=w851) -> ("instrument handle"=w854:refnum<k15>, "error out"=w853:errorcluster)  [unwired: 11 in]
            }
            n155 = property on="Trigger Source Window" class="CmbBox (strict)"("Value"=T4 "0" ("Trigger Source Edge")) -> ()  [unwired: 2 in, 2 out]
          }
          frame "3" {
            n156 = for {
              tunnel: w858 -> [w863] mode=indexing
              shift-right: [w865] -> w861
              shift-left: w857 -> [w864]
              # "13"
              n157 = call <instrlib>:"niScope Close.vi"("instrument handle"=w863, "error in"=w864) -> ("error out"=w865:errorcluster)  [unwired: 13 in]
            }
            n158 = for {
              tunnel: [w869] -> w859 mode=indexing
              shift-right: [w868] -> w860
              shift-left: w861 -> [w866]
              tunnel: refnum<k15>[] ["Dev2", "Dev1"] ("Resources") -> [w867] mode=indexing
              w870 = FALSE  # reset device
              # "1"
              n159 = call <instrlib>:"niScope Initialize.vi"("resource name"=w867, "reset device"=w870, "error in"=w866) -> ("instrument handle"=w869:refnum<k15>, "error out"=w868:errorcluster)  [unwired: 11 in]
            }
            n160 = property on="Trigger Source Window" class="CmbBox (strict)"("Value"=T4 "1" ("Trigger Source Edge")) -> ()  [unwired: 2 in, 2 out]
          }
        }
      }
    }
    "Array" <- w377
    n161 = event shown="[0] Timeout" {
      selector: _ -> [_ _]
      dyn-events: _ -> [_ _]
      timeout: 1 -> [_ _]
      event Timeout {
        n162 = event-data() -> ()  [unwired: 1 in, 2 out]
      }
      event "Trigger": Value Change {
        n163 = event-data() -> ("NewVal"=w670:T3)  [unwired: 1 in, 4 out]
        n164 = case shown="\"Edge\"" w670 {
          frame "Immediate", Default {
          }
          frame "Edge" {
            n165 = property on="Trigger Source Edge 2" class="CmbBox (strict)"() -> ("Value"=w671:T4)  [unwired: 2 in, 2 out]
            n166 = property on="Trigger Source Edge 2" class="CmbBox (strict)"("Val(Sgnl)"=w671) -> ()  [unwired: 2 in, 2 out]
          }
          frame "Window" {
            n167 = property on="Trigger Source Window 2" class="CmbBox (strict)"() -> ("Value"=w672:T4)  [unwired: 2 in, 2 out]
            n168 = property on="Trigger Source Window 2" class="CmbBox (strict)"("Val(Sgnl)"=w672) -> ()  [unwired: 2 in, 2 out]
          }
          frame "Hysteresis" {
            n169 = property on="Hysteresis Source Trigger 2" class="CmbBox (strict)"() -> ("Value"=w673:T4)  [unwired: 2 in, 2 out]
            n170 = property on="Hysteresis Source Trigger 2" class="CmbBox (strict)"("Val(Sgnl)"=w673) -> ()  [unwired: 2 in, 2 out]
          }
        }
      }
    }
    n171 = for {
      tunnel: w377 -> [w904] mode=indexing
      shift-right: [w882] -> w389
      shift-left: w378 -> [w903]
      tunnel: w382 -> [w895]
      tunnel: "Min Sample Rate" -> [w888]
      tunnel: "Trigger" -> [w887]
      tunnel: "Bandwidth" -> [w885]
      tunnel: "Reference Position (%)" -> [w884]
      tunnel: [w881] -> w371 mode=indexing
      tunnel: [w880] -> w386 mode=indexing
      tunnel: ["Min Record Length"] -> w370
      i -> [w889]
      w877 = u32 0 items=["1 mega ohm"] ("input impedance")
      w902 = TRUE  # Enforce Realtime
      n172 = call <instrlib>:"niScope Configure Acquisition.vi"("instrument handle"=w904, "error in"=w903) -> ("instrument handle out"=w900:refnum<k15>, "error out"=w901:errorcluster)  [unwired: 12 in]
      n173 = call <instrlib>:"niScope Configure Vertical.vi"("instrument handle"=w900, "probe attenuation"="Probe Attenuation", "vertical coupling"="Vertical Coupling", "channels"=w895, "vertical range"="Vertical Range", "vertical offset"="Vertical Offset", "error in"=w901) -> ("instrument handle out"=w899:refnum<k15>, "error out"=w898:errorcluster)  [unwired: 7 in]
      n174 = call <instrlib>:"niScope Configure Chan Characteristics.vi"("instrument handle"=w899, "channels"=w895, "input impedance"=w877, "maximum input frequency"=w885, "error in"=w898) -> ("instrument handle out"=w896:refnum<k15>, "error out"=w897:errorcluster)  [unwired: 9 in]
      n175 = call <instrlib>:"niScope Configure Horizontal Timing.vi"("instrument handle"=w896, "enforce realtime"=w902, "min sample rate"=w888, "reference position"=w884, "error in"=w897, "min record length"="Min Record Length") -> ("instrument handle out"=w891:refnum<k15>, "error out"=w892:errorcluster)  [unwired: 8 in]
      n176 = case shown="0" w889 {
        tunnel: w892 -> [w905 w911]
        tunnel: w891 -> [w906 w910]
        tunnel: [w906 w909] -> w879
        tunnel: [w905 w908] -> w883
        tunnel: w887 -> [_ w907]
        frame 1, Default {
        }
        frame 0 {
          # "6"
          n177 = case "Trigger Selection" shown="\"Edge\"" w907 {
            tunnel: w911 -> [w920 w930 w940 w944]
            tunnel: [w917 w927 w937 w941] -> w908
            tunnel: w910 -> [w919 w929 w939 w943]
            tunnel: [w918 w928 w938 w942] -> w909
            frame "Edge" {
              n178 = call-poly <instrlib>:"niScope Configure Trigger (poly).vi"("instrument handle"=w919, "trigger slope"="Slope", "trigger coupling"="Coupling", "trigger source"="Trigger Source Edge", "trigger level"="Level", "error in"=w920, "trigger delay"="Delay") -> ("instrument handle out"=w918:refnum<k15>, "error out"=w917:errorcluster)  [unwired: 7 in]
            }
            frame "Hysteresis" {
              n179 = call-poly <instrlib>:"niScope Configure Trigger (poly).vi"("instrument handle"=w929, "trigger slope"="Slope", "trigger coupling"="Hysteresis Coupling", "trigger source"="Hysteresis Source Trigger", "trigger level"="Level", "hysteresis"="Hysteresis", "error in"=w930, "trigger delay"="Delay") -> ("instrument handle out"=w928:refnum<k15>, "error out"=w927:errorcluster)  [unwired: 6 in]
            }
            frame "Window" {
              n180 = call-poly <instrlib>:"niScope Configure Trigger (poly).vi"("instrument handle"=w939, "trigger window mode"="Window Mode", "trigger coupling"="Window Coupling", "trigger source"="Trigger Source Window", "low level"="Low Level", "high level"="High Level", "error in"=w940, "trigger delay"="Delay") -> ("instrument handle out"=w938:refnum<k15>, "error out"=w937:errorcluster)  [unwired: 6 in]
            }
            frame "Immediate", Default {
              n181 = call-poly <instrlib>:"niScope Configure Trigger (poly).vi"("instrument handle"=w943, "error in"=w944) -> ("instrument handle out"=w942:refnum<k15>, "error out"=w941:errorcluster)  [unwired: 12 in]
            }
          }
        }
      }
      n182 = call <instrlib>:"niScope Get Session Reference.vi"("instrument handle"=w879, "error in"=w883) -> ("instrument handle out"=w881:refnum<k15>, "session reference"=w880:refnum<k20>, "error out"=w882:errorcluster)  [unwired: 11 in]
    }
    n183 = Bundle(cluster=w393, "Trigger", "Min Sample Rate", "Reference Position (%)", "Bandwidth") -> (w392:cluster{i32, dbl, dbl, dbl})
    n184 = Not Equal?(x=w393, y=w392) -> (x != y?=w360:bool)
    n185 = property on="Trigger Source Edge" class="CmbBox (strict)"("Visible"="Debug Mode\n(Confusing)") -> ()  [unwired: 2 in, 2 out]
    n186 = property on="Hysteresis Source Trigger" class="CmbBox (strict)"("Visible"="Debug Mode\n(Confusing)") -> ()  [unwired: 2 in, 2 out]
    n187 = property on="Trigger Source Window" class="CmbBox (strict)"("Visible"="Debug Mode\n(Confusing)") -> ()  [unwired: 2 in, 2 out]
    n188 = call <instrlib>:"niTClk Configure For Homogeneous Triggers.vi"("error in (no error)"=w389, "sessions"=w386) -> ("error out"=w388:errorcluster, "sessions out"=w387:refnum<k20>[])  [unwired: 8 in]
    n189 = case shown="False" w360 {
      tunnel: [w874 w876] -> w398
      tunnel: [w873 w875] -> w397
      tunnel: w387 -> [w871 w876]
      tunnel: w388 -> [w872 w875]
      frame True {
        n190 = call <instrlib>:"niTClk Synchronize.vi"("error in (no error)"=w872, "sessions"=w871) -> ("error out"=w873:errorcluster, "sessions out"=w874:refnum<k20>[])  [unwired: 8 in]
      }
      frame False {
      }
    }
    n191 = call <instrlib>:"niTClk Initiate.vi"("error in (no error)"=w397, "sessions"=w398) -> ("error out"=w399:errorcluster)  [unwired: 8 in, 1 out]
    n192 = event shown="[0] Timeout" {
      selector: _ -> [_ _ _]
      dyn-events: _ -> [_ _ _]
      timeout: 1 -> [_ _ _]
      tunnel: [w628 w645 w661] -> w376
      tunnel: [w627 w644 w660] -> w375
      tunnel: [w626 w643 w659] -> w374
      tunnel: [w625 w642 w658] -> w373
      tunnel: w371 -> [w623 _ _]
      tunnel: "Debug Mode\n(Confusing)" -> [w619 w640 w655]
      event Timeout {
        n193 = event-data() -> ()  [unwired: 1 in, 2 out]
        n194 = Equal?(x=w623, y=refnum<k15>[] ["Dev1", "Dev2"] ("Resources")) -> (x = y?=w622:bool[])
        n195 = And Array Elements(Boolean array=w622) -> (logical AND=w620:bool)
        n196 = Or(x=w619, y=w620) -> (x .or. y?=w621:bool)
        n197 = case shown="False" w621 {
          tunnel: [2 ("index") 0 ("index")] -> w628
          tunnel: [3 ("index") 1 ("index")] -> w627
          tunnel: [0 ("index") 2 ("index")] -> w626
          tunnel: [1 ("index") 3 ("index")] -> w625
          frame False {
          }
          frame True {
          }
        }
      }
      event Value Change {
        n198 = event-data() -> ("NewVal"=w637:T2)  [unwired: 1 in, 4 out]
        n199 = Equal?(x=w637, y=refnum<k15>[] ["Dev1", "Dev2"] ("Resources")) -> (x = y?=w646:bool[])
        n200 = And Array Elements(Boolean array=w646) -> (logical AND=w639:bool)
        n201 = Or(x=w640, y=w639) -> (x .or. y?=w638:bool)
        n202 = case shown="True" w638 {
          tunnel: [2 ("index") 0 ("index")] -> w645
          tunnel: [3 ("index") 1 ("index")] -> w644
          tunnel: [0 ("index") 2 ("index")] -> w643
          tunnel: [1 ("index") 3 ("index")] -> w642
          frame False {
          }
          frame True {
          }
        }
      }
      event "Debug Mode\n(Confusing)": Value Change {
        n203 = event-data() -> ("NewVal"=w656:bool)  [unwired: 1 in, 4 out]
        n204 = Or(x=w656, y=w655) -> (x .or. y?=w657:bool)
        n205 = case shown="True" w657 {
          tunnel: [2 ("index") 0 ("index")] -> w661
          tunnel: [3 ("index") 1 ("index")] -> w660
          tunnel: [0 ("index") 2 ("index")] -> w659
          tunnel: [1 ("index") 3 ("index")] -> w658
          frame False {
          }
          frame True {
          }
        }
      }
    }
    n206 = for {
      tunnel: w382 -> [w614]
      tunnel: w371 -> [w610] mode=indexing
      shift-right: [w618] -> w361
      shift-left: T13 [] ("Waveform Graph") -> [w612]
      shift-right: [w601] -> w354
      shift-left: w399 -> [w611]
      tunnel: w370 -> [_]
      tunnel: [w603] -> w359 mode=indexing
      tunnel: [w609] -> w363
      n207 = call-poly <instrlib>:"niScope Fetch (poly).vi"("timeout"=1.0 ("Timeout (s)"), "error in"=w611, "channels"=w614, "instrument handle"=w610) -> ("error out"=w605:errorcluster, "waveform"=w613:T19, "instrument handle out"=w606:refnum<k15>)  [unwired: 4 in, 1 out]
      "error out 2" <- w605
      n208 = call <instrlib>:"niScope Actual Record Length.vi"("instrument handle"=w606, "error in"=w605) -> ("instrument handle out"=w617:refnum<k15>, "actual record length"=→"Actual Record Length":i32, "error out"=w616:errorcluster)  [unwired: 11 in]
      n209 = call <instrlib>:"niScope Sample Rate.vi"("instrument handle"=w617, "error in"=w616) -> ("instrument handle out"=w604:refnum<k15>, "actual sample rate"=→"Actual Sample Rate":dbl, "error out"=w602:errorcluster)  [unwired: 11 in]
      n210 = Get Date/Time In Seconds() -> (seconds since 1Jan1904=w609:timestamp)
      n211 = Build Array (concatenate)(w612, w613) -> (w618:T19)
      n212 = call <instrlib>:"niScope Abort.vi"("instrument handle"=w604, "error in"=w602) -> ("instrument handle out"=w603:refnum<k15>, "error out"=w601:errorcluster)  [unwired: 12 in]
    }
    n213 = case shown="No Error" w354 {
      tunnel: [w476 w593] -> w385
      tunnel: [w475 w594] -> w384
      tunnel: w383 -> [w474 w594]
      tunnel: w376 -> [w472 _]
      tunnel: w375 -> [w471 _]
      tunnel: w374 -> [w470 _]
      tunnel: w373 -> [w469 _]
      tunnel: w369 -> [w462 _]
      tunnel: w368 -> [w461 _]
      tunnel: [w456 w595] -> w367
      tunnel: w366 -> [w455 w595]
      tunnel: w363 -> [w404 _]
      tunnel: w362 -> [w441 w593]
      tunnel: w361 -> [w431 _]
      tunnel: w354 -> [w426 w592]
      tunnel: [w402 w592] -> w352
      tunnel: w351 -> [w410 w591]
      tunnel: w350 -> [w414 _]
      tunnel: w349 -> [w413 w590]
      tunnel: [w412 w590] -> w348
      tunnel: [w411 w591] -> w347
      tunnel: w346 -> [w407 w589]
      tunnel: [w406 w589] -> w345
      frame No Error {
        w464 = 12100000000000.0 ("x")
        # "Make Sure 50Ohm"
        n214 = Increment(x=w407) -> (x+1=w408:dbl)
        n215 = String To Path(string="Location") -> (path=w459:path)
        n216 = event shown="[0] Timeout" {
          selector: _ -> [_ _]
          dyn-events: _ -> [_ _]
          timeout: 1 -> [_ _]
          tunnel: w459 -> [w544 w558]
          tunnel: [w539 w555] -> w443
          tunnel: w455 -> [w538 w554]
          tunnel: [w537 w553] -> w454
          event Timeout {
            n217 = event-data() -> ()  [unwired: 1 in, 1 out]
            n218 = local read "Write Metadata?"() -> (w535:bool)
            n219 = local read "Write Raw File?"() -> (w536:bool)
            n220 = call <vilib>:"Check if File or Folder Exists.vi"("path"=w544) -> ("file or folder exists?"=w543:bool, "dup path"=w540:path)  [unwired: 8 in, 1 out]
            n221 = Not(x=w543) -> (.not. x?=w542:bool)
            n222 = Or(x=w536, y=w535) -> (x .or. y?=w534:bool)
            n223 = And(x=w542, y=w534) -> (x .and. y?=w541:bool)
            n224 = case shown="True" w541 {
              tunnel: [w546 w549] -> w539
              tunnel: w540 -> [w546 w548]
              tunnel: w538 -> [w545 _]
              tunnel: [w545 0] -> w537
              frame False {
              }
              frame True {
                n225 = Create Folder(path (use dialog)=w548) -> (created path=w549:path)  [unwired: 2 in, 2 out]
              }
            }
          }
          event "Write Raw File?", "Location", "Write Metadata?": Value Change {
            n226 = event-data() -> ()  [unwired: 1 in, 1 out]
            n227 = local read "Write Metadata?"() -> (w551:bool)
            n228 = local read "Write Raw File?"() -> (w552:bool)
            n229 = call <vilib>:"Check if File or Folder Exists.vi"("path"=w558) -> ("file or folder exists?"=w557:bool, "dup path"=w556:path)  [unwired: 8 in, 1 out]
            n230 = Not(x=w557) -> (.not. x?=w560:bool)
            n231 = Or(x=w552, y=w551) -> (x .or. y?=w550:bool)
            n232 = And(x=w560, y=w550) -> (x .and. y?=w559:bool)
            n233 = case shown="True" w559 {
              tunnel: [w562 w565] -> w555
              tunnel: w556 -> [w562 w564]
              tunnel: w554 -> [w561 _]
              tunnel: [w561 0] -> w553
              frame False {
              }
              frame True {
                n234 = Create Folder(path (use dialog)=w564) -> (created path=w565:path)  [unwired: 2 in, 2 out]
              }
            }
          }
        }
        "created path" <- w443
        n235 = Add(x=w408, y=0.0) -> (x+y=w406:dbl)
        "Acquisition #" <- w406
        n236 = Index Array(array=w431, index #1=w472, index #2=w471, index #3=w470, index #4=w469) -> (element #1=w430:T20, element #2=w429:T20, element #3=w428:T20, element #4=w427:T20)
        n237 = Build Array(w430, w429, w428, w427) -> (w405:T13)
        n238 = Tick Count (ms)() -> (millisecond timer value=w419:u32)
        n239 = Unbundle(w430) -> ("xIncrement"=w451:dbl, "Waveforms"=w440:dbl[])  [unwired: 1 out]
        n240 = Unbundle(w429) -> ("Waveforms"=w439:dbl[])  [unwired: 2 out]
        n241 = Unbundle(w428) -> ("Waveforms"=w438:dbl[])  [unwired: 2 out]
        n242 = Unbundle(w427) -> ("Waveforms"=w437:dbl[])  [unwired: 2 out]
        n243 = Subtract(x=w419, y=w414) -> (x-y=w411:u32)
        n244 = Subtract(x=w411, y=w410) -> (x-y=w420:u32)
        n245 = event shown="[1] \"Write Metadata?\": Value Change" {
          selector: _ -> [_ _]
          dyn-events: _ -> [_ _]
          timeout: 1 -> [_ _]
          tunnel: [w502 w514] -> w444
          tunnel: w443 -> [w501 w515]
          event Timeout {
            n246 = event-data() -> ()  [unwired: 1 in, 2 out]
            n247 = local read "Write Metadata?"() -> (w497:bool)
            n248 = local read "Acquisition #"() -> (w500:i32)
            n249 = Equal To 0?(x=w500) -> (x = 0?=w498:bool)
            n250 = And(x=w498, y=w497) -> (x .and. y?=w499:bool)
            n251 = case shown="True" w499 {
              tunnel: [w503 w505] -> w502
              tunnel: w501 -> [_ w504]
              frame False {
                n252 = local read "Metadata Path"() -> (w503:path)
              }
              frame True {
                n253 = Get Date/Time In Seconds() -> (seconds since 1Jan1904=w508:timestamp)
                n254 = Format Date/Time String(time format string (%c)="%Y%m%d%H%M%S", seconds (now)=w508) -> (date/time string=w512:string)  [unwired: 1 in]
                n255 = Path To String(path=w504) -> (string=w506:string)
                n256 = Concatenate Strings(w506, "\\" ("string"), w512, ".csv") -> (w510:string)
                n257 = String To Path(string=w510) -> (path=w505:path)
              }
            }
          }
          event "Write Metadata?": Value Change {
            n258 = event-data() -> ()  [unwired: 1 in, 1 out]
            n259 = local read "Write Metadata?"() -> (w513:bool)
            n260 = case shown="True" w513 {
              tunnel: w515 -> [w516 w518]
              tunnel: [w516 w517] -> w514
              frame False {
              }
              frame True {
                n261 = Get Date/Time In Seconds() -> (seconds since 1Jan1904=w521:timestamp)
                n262 = Format Date/Time String(time format string (%c)="%Y%m%d%H%M%S", seconds (now)=w521) -> (date/time string=w525:string)  [unwired: 1 in]
                n263 = Path To String(path=w518) -> (string=w519:string)
                n264 = Concatenate Strings(w519, "\\" ("string"), w525, ".csv") -> (w523:string)
                n265 = String To Path(string=w523) -> (path=w517:path)
              }
            }
          }
        }
        "Metadata Path" <- w444
        n266 = Rotate 1D Array(1:w413, 2:1 ("n")) -> (0:w423:dbl[])
        n267 = Bundle By Name("t0"=w404, "Y"=w440, "dt"=w451) -> (w468:waveform(dbl))  [unwired: 1 in]
        n268 = Bundle By Name("Y"=w439, "dt"=w451) -> (w467:waveform(dbl))  [unwired: 1 in]
        n269 = Bundle By Name("Y"=w438, "dt"=w451) -> (w466:waveform(dbl))  [unwired: 1 in]
        "Charge Detector/PSU gate (CH2)" <- w466
        n270 = Bundle By Name("Y"=w437, "dt"=w451) -> (w465:waveform(dbl))  [unwired: 1 in]
        "Final Detector (CH3)" <- w465
        n271 = Divide(x=w420, y=1000.0) -> (x/y=w418:dbl)
        "Time Between Triggers" <- w418
        n272 = Replace Array Subset(array=w423, new element=w418, index=0) -> (w412:dbl[])
        n273 = Array Max & Min(array=w439) -> (min index (indices)=w453:i32)  [unwired: 3 out]
        n274 = Array Max & Min(array=w440) -> (min index (indices)=w452:i32)  [unwired: 3 out]
        n275 = call-poly <vilib>:"Mean.vi"("X"=w412) -> ("mean"=w417:dbl)  [unwired: 1 out]
        n276 = Subtract(x=w453, y=w452) -> (x-y=w489:i32)
        n277 = Build Array(w468, w467) -> (→"Velocity Detectors (CH0 & CH1)":waveform(dbl)[])
        n278 = Divide(x=0.6, y=w489) -> (x/y=w487:dbl)
        n279 = Divide(x=w487, y=w451) -> (x/y=w485:dbl)
        n280 = Reciprocal(x=w417) -> (1/x=→"Average Frequency":dbl)
        n281 = Bundle("mean"=w417, "Ideal Time (Cursor)"="Ideal Time (Cursor)") -> (→"?":cluster{"mean":dbl, "Ideal Time (Cursor)":dbl})  [unwired: 1 in]
        n282 = call "Filter"("error in (no error)"=w426, "Signal"=w465) -> ("error out"=w450:errorcluster, "Filtered Signal"=w473:dynamicdata)  [unwired: 8 in]
        n283 = Greater?(x=w485, y=0.0 ("x")) -> (0:w486:bool)
        n284 = case shown="False" w486 {
          tunnel: w485 -> [_ w588]
          tunnel: [w587 w588] -> w433
          frame False {
            w587 = 500.0 ("Velocity")
            n285 = property on="Velocity (Est.)" class="DigNum (strict)"("Value"=w587) -> ()  [unwired: 2 in, 2 out]
          }
          frame True {
            "Velocity (Est.)" <- w588
          }
        }
        n286 = Build Array(w468, w467, w466, w465) -> (w436:waveform(dbl)[])
        n287 = call "Convert from Dynamic Data"("Dynamic Data Type"=w473) -> ("Array"=w483:dbl[])  [unwired: 3 in]
        n288 = Array Max & Min(array=w483) -> (min value=w482:dbl)  [unwired: 3 out]
        n289 = Reciprocal(x=w464) -> (1/x=w463:dbl)
        n290 = Absolute Value(x=w482) -> (abs(x)=w481:dbl)
        n291 = Multiply(x="Acceleration Voltage (MV)", y=1000000.0) -> (x*y=w445:dbl)
        n292 = Multiply(x=w481, y=w463) -> (x*y=w434:dbl)
        "Charge" <- w434
        n293 = Multiply(x=w445, y=w434) -> (x*y=w480:dbl)
        n294 = case shown="True" "Write Raw File?" {
          tunnel: w436 -> [_ w570]
          tunnel: [w567 w584] -> w401
          tunnel: w450 -> [w569 w582]
          tunnel: w462 -> [_ w571]
          tunnel: w461 -> [w568 w580]
          tunnel: w443 -> [_ w578]
          tunnel: [w566 w576] -> w456
          tunnel: w454 -> [w566 w575]
          frame False {
            n295 = Merge Errors(w568, w569) -> (w567:errorcluster)
          }
          frame True {
            n296 = Path To String(path=w578) -> (string=w573:string)
            n297 = Format Value(format string="%05.0", value (0)=w575) -> (output string=w577:string)  [unwired: 1 in]
            n298 = Concatenate Strings(w573, "\\" ("string"), "WFM Tag", w577) -> (w586:string)
            n299 = String To Path(string=w586) -> (path=w579:path)
            n300 = Bundle(w579, w570) -> (w581:cluster{path, waveform(dbl)[]})  [unwired: 1 in]
            "output cluster" <- w581
            n301 = Merge Errors(w580, w582) -> (w583:errorcluster)
            n302 = Enqueue Element(queue=w571, element=w581, error in (no error)=w583) -> (error out=w584:errorcluster)  [unwired: 1 in, 2 out]
            n303 = Increment(x=w575) -> (x+1=w576:i32)
          }
        }
        n304 = Square(x=w433) -> (x^2=w479:dbl)
        n305 = Divide(x=w480, y=w479) -> (x/y=w435:dbl)
        "Mass" <- w435
        n306 = Format Into String(format string="%5.2f,%.2e,%.2e,%2.1f", w433, w435, w434, "Acceleration Voltage (MV)") -> (resulting string=w447:string)  [unwired: 2 in, 1 out]
        n307 = case shown="False" "Write Metadata?" {
          tunnel: w447 -> [_ w529]
          tunnel: w444 -> [_ w526]
          frame False {
          }
          frame True {
            n308 = Get Date/Time In Seconds() -> (seconds since 1Jan1904=w533:timestamp)
            n309 = Format Date/Time String(time format string (%c)="%Y%m%d%H%M%S%2u", seconds (now)=w533) -> (date/time string=w531:string)  [unwired: 1 in]
            n310 = Build Array(w531, "," ("string"), w529) -> (w527:string[])
            n311 = call-poly <vilib>:"Write To Spreadsheet File.vi"("append to file? (new file:F)"=TRUE, "1D data"=w527, "file path (dialog if empty)"=w526) -> ()  [unwired: 5 in, 1 out]
          }
        }
        n312 = Build Array (concatenate)(w441, w433) -> (w476:dbl[])
        n313 = Build Array (concatenate)(w474, w435) -> (w475:dbl[])
        n314 = Bundle By Name(cluster=T14 {"Time Stamp"=timestamp(0 s since 1904-01-01), "Velocity"=0.0, "Mass"=0.0, "Charge"=0.0, "Radius"=0.0, "Array"=[], "Dust Event ID"=0, "Passed_3rd_Detector"=FALSE, "Estimate Source"=0, "Estimate Quality"=0.0} ("Input Data"), "Velocity"=w433, "Mass"=w435, "Charge"=w434) -> (w403:T14)
        n315 = case shown="True" "Write to Database?" {
          tunnel: w405 -> [_ w496]
          tunnel: w404 -> [_ w495]
          tunnel: w403 -> [_ w494]
          tunnel: [w491 w493] -> w402
          tunnel: w401 -> [w491 w492]
          frame False {
          }
          frame True {
            n316 = call "Call_enqueue.vi"("Waveform"=w496, "error in"=w492, "Input Data"=w494, "seconds since 1Jan1904"=w495) -> ("error IO"=w493:errorcluster)  [unwired: 7 in]
          }
        }
        n317 = Bundle "Bundle"(w476, w475) -> (→"Multi Plot 2":cluster{dbl[], dbl[]})  [unwired: 1 in]
        "Calibration" <- w464
      }
      frame Error {
      }
    }
    n318 = case shown="True" "Limit Triggers" {
      tunnel: [FALSE w599] -> w356
      frame False {
      }
      frame True {
        n319 = local read "Acquisition #"() -> (w598:i32)
        n320 = Decrement(x="Limit") -> (x-1=w597:dbl)
        n321 = Equal?(x=w597, y=w598) -> (x = y?=w599:bool)
      }
    }
    n322 = Or(x=w356, y="stop") -> (x .or. y?=w357:bool)
    "Stop condition" <- w357
    n323 = call <vilib>:"Clear Errors.vi"("error in (no error)"=w352) -> ("error out"=w353:errorcluster)  [unwired: 6 in]
  }
  n324 = Obtain Queue(name (unnamed)=w18, element data type=w17, error in (no error)=w16) -> (queue out=w24:refnum<queue>, error out=w23:errorcluster)  [unwired: 2 in, 1 out]
  n325 = while {
    tunnel: w24 -> [w952]
    tunnel: w23 -> [w945]
    tunnel: [w961] -> w22
    tunnel: [w959] -> w21
    i -> [w955]
    stop <- w958 stop-if-true
    n326 = local read "Stop condition"() -> (w947:bool)
    n327 = local read "Write Raw File?"() -> (w949:bool)
    n328 = Get Queue Status(queue=w952, error in (no error)=w945) -> (queue out=w946:refnum<queue>, error out=w953:errorcluster, # elements in queue=w951:i32)  [unwired: 1 in, 5 out]
    "# elements in queue" <- w951
    n329 = And(x=w949, y=w947) -> (x .and. y?=w960:bool)
    n330 = Not Equal To 0?(x=w951) -> (x != 0?=w950:bool)
    n331 = property on="Saving Raw File..." class="Path"("Blinking"=w960) -> ()  [unwired: 2 in, 2 out]
    n332 = And(x=w950, y=w949) -> (x .and. y?=w954:bool)
    n333 = local read "Stop condition"() -> (w948:bool)
    n334 = case shown="True" w954 {
      tunnel: w946 -> [w965 w984]
      tunnel: [w963 w982] -> w959
      tunnel: [w964 w980] -> w961
      tunnel: w948 -> [w966 w979]
      tunnel: [w966 w976] -> w956
      tunnel: w953 -> [w962 w972]
      frame False {
        n335 = Flush Queue(queue=w965, error in (no error)=w962) -> (queue out=w964:refnum<queue>, error out=w963:errorcluster)  [unwired: 1 out]
      }
      frame True {
        n336 = Dequeue Element(queue=w984, error in (no error)=w972) -> (queue out=w981:refnum<queue>, element=w983:cluster{path, waveform(sgl)[]}, error out=w970:errorcluster)  [unwired: 1 in, 1 out]
        n337 = Unbundle(w983) -> (w971:path, w967:waveform(sgl)[])
        n338 = Get Queue Status(queue=w981, error in (no error)=w970) -> (queue out=w980:refnum<queue>, error out=w969:errorcluster, # elements in queue=w978:i32)  [unwired: 1 in, 5 out]
        n339 = Equal To 0?(x=w978) -> (x = 0?=w977:bool)
        n340 = call <vilib>:"Check if File or Folder Exists.vi"("error in (no error)"=w969, "path"=w971) -> ("error out"=w968:errorcluster, "file or folder exists?"=w975:bool, "dup path"=w974:path)  [unwired: 7 in]
        n341 = case shown="True" w975 {
          tunnel: w974 -> [w985 _]
          tunnel: [w985 w991] -> w973
          frame False {
          }
          frame True {
            n342 = local read "created path"() -> (w988:path)
            n343 = local read "WFM Tag"() -> (w993:string)
            n344 = File/Directory Info(path=w988) -> (size=w989:i64)  [unwired: 1 in, 6 out]
            n345 = Format Value(format string="%05.0", value (0)=w989) -> (output string=w992:string)  [unwired: 1 in]
            n346 = Path To String(path=w988) -> (string=w986:string)
            n347 = Concatenate Strings(w986, "\\" ("string"), w993, w992) -> (w990:string)
            n348 = String To Path(string=w990) -> (path=w991:path)
          }
        }
        "Saving Raw File..." <- w973
        n349 = And(x=w977, y=w979) -> (x .and. y?=w976:bool)
        n350 = Write to Binary File(file (use dialog)=w973, data=w967, error in=w968) -> (error out=w982:errorcluster)  [unwired: 3 in, 2 out]
      }
    }
    n351 = Unbundle By Name(w959) -> ("status"=w957:bool)
    n352 = Or(x=w956, y=w957) -> (x .or. y?=w958:bool)
    "Numeric" <- w955
  }
  n353 = Release Queue(queue=w22, error in (no error)=w21) -> (error out=w7:errorcluster)  [unwired: 1 in, 2 out]
  n354 = call <vilib>:"Clear Errors.vi"("error in (no error)"=w7) -> ("error out"=w6:errorcluster)  [unwired: 6 in]
  n355 = Merge Errors(w6, w12, w1) -> (w8:errorcluster)
  n356 = for {
    tunnel: w27 -> [w995] mode=indexing
    shift-right: [w997] -> w39
    shift-left: w8 -> [w996]
    # "13"
    n357 = call <instrlib>:"niScope Close.vi"("instrument handle"=w995, "error in"=w996) -> ("error out"=w997:errorcluster)  [unwired: 13 in]
  }
  n358 = call <vilib>:"General Error Handler.vi"("type of dialog (OK msg:1)"=w9, "error in (no error)"=w39) -> ("message"=w35:string, "error out"=w37:errorcluster)  [unwired: 9 in, 3 out]
  n359 = Bundle By Name(cluster=w37, "source"=w35) -> (→"error out":errorcluster)
